vi "GetText.vi"(8 "error in":errorcluster, 11 "cRIO in":refnum<class "cRIO  node root.lvclass">) -> (0 "error out":errorcluster, 1 "additional text":string, 2 "text":string, 3 "cRIO out":refnum<class "cRIO  node root.lvclass">, 4 "glyph":string)   [LabVIEW 2013, in "cRIO  node root.lvclass"]
uses:
  cRIO  node root.lvclass
  cRIO  node root.lvclass/cRIO  node root.ctl
  CEF_TreeControl/serializable configuration/read metadata property.vi
  crio configuration/crio configuration.lvclass
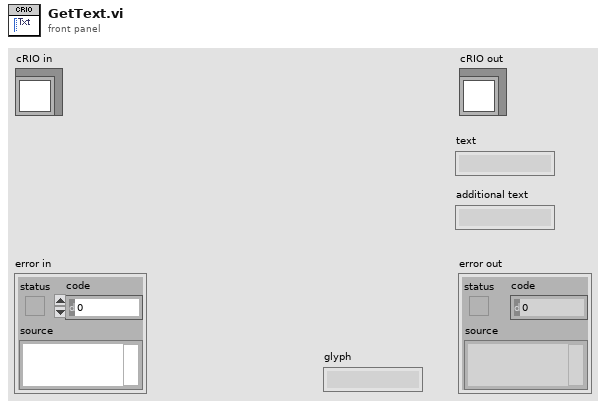
[diagram p1: front panel]
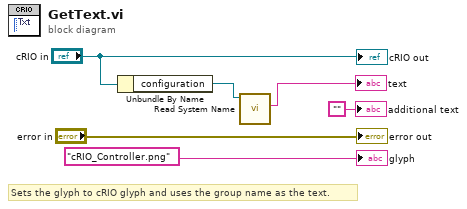
[diagram p0: block diagram]
diagram:
  # "Sets the glyph to cRIO glyph and uses the group name as the text."
  n1 = Unbundle By Name("cRIO in") -> ("configuration"=w2:refnum<class "cRIO configuration.lvclass">)
  n2 = call "Read System Name.vi"("crio configuration in"=w2) -> ("System Name"=→"text":string)  [unwired: 8 in, 2 out]
  "error out" <- "error in"
  "cRIO out" <- "cRIO in"
  "additional text" <- ""
  "glyph" <- "cRIO_Controller.png" ("glyph")
